vi "Memory.Array.Set Number of Elements.vi"(8 "error in (no error)":errorcluster, 10 "number of elements":u64, 11 "Memory.Array in":refnum<class "Memory.Array.lvclass">) -> (0 "error out":errorcluster, 3 "Memory.Array out":refnum<class "Memory.Array.lvclass">)   [LabVIEW 2016, in "LabVIEW Memory Manager.lvlib" / "Memory.Array.lvclass"]
uses:
  Memory.Array.lvclass
  Memory.Array.lvclass/Memory.Array.ctl
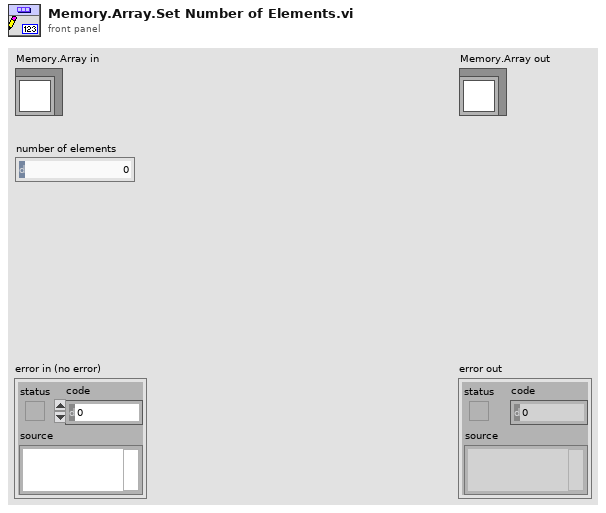
[diagram p1: front panel]
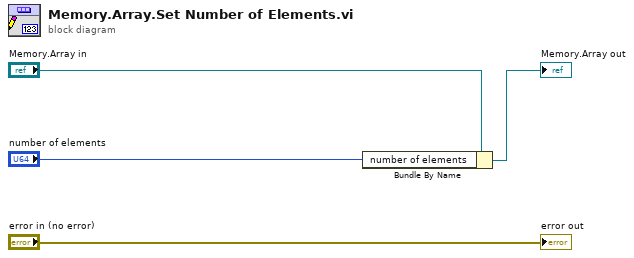
[diagram p0: block diagram]
diagram:
  n1 = Bundle By Name(cluster="Memory.Array in", "number of elements"="number of elements") -> (→"Memory.Array out":refnum<class "Memory.Array.lvclass">)
  "error out" <- "error in (no error)"
